vi "ExSubSetInitCamSameGraph.vi"(2 "error in (no error)":errorcluster, 3 "Exposure":dbl min=0.0 step=0.001 format="%.3f", 4 "Camera Handle":u32) -> (0 "error out":errorcluster, 1 "Camera Handle 2":u32)   [LabVIEW 2010]
panel:
  # "ExSubSetInitCam:\nThis sub vi initializes the camera."
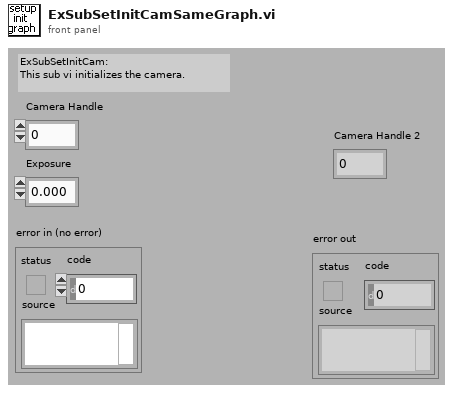
[diagram p1: front panel]
types:
  T1 = cluster{"acquire focus mode":u32, "Exposure":dbl, "Number of Images":u32, "Software accumulation":u32}
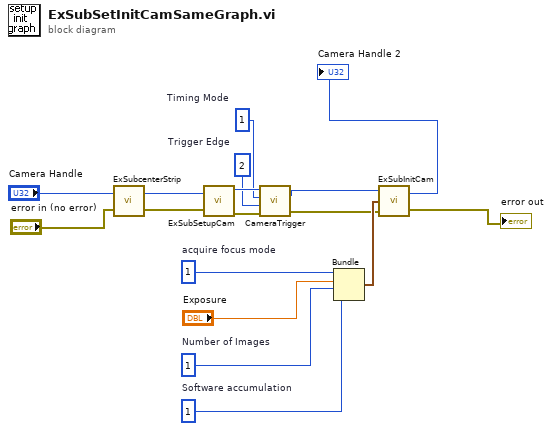
[diagram p0: block diagram]
diagram:
  w9 = u32 1  # Timing Mode
  w10 = u32 2  # Trigger Edge
  w13 = u32 1  # acquire focus mode
  w12 = u32 1  # Number of Images
  w11 = u32 1  # Software accumulation
  n1 = call "ExSubcenterStrip.vi"("error in (no error)"="error in (no error)", "Camera Handle"="Camera Handle") -> ("error out"=w5:errorcluster, "Camera Handle"=w4:u32)
  n2 = call "ExSubSetupCam.vi"("error in (no error)"=w5, "Camera Handle"=w4) -> ("error out"=w14:errorcluster, "Camera Handle"=w15:u32)
  n3 = call <userlib>:"CameraTrigger.vi"("error in"=w14, "Trigger Edge"=w10, "Timing Mode"=w9, "Camera Handle"=w15) -> ("error out"=w7:errorcluster, "Camera Handle"=w8:u32)
  n4 = Bundle("acquire focus mode"=w13, "Exposure"="Exposure", "Number of Images"=w12, "Software accumulation"=w11) -> (w16:T1)  [unwired: 1 in]
  n5 = call "ExSubInitCam.vi"("error in (no error)"=w7, "Camera Information"=w16, "Camera Handle"=w8) -> ("error out"=→"error out":errorcluster, "Camera Handle"=→"Camera Handle 2":u32)
